vi "RUSHTarget.vi"(8 "Turret Case":i32, 9 "Joystick Value":dbl, 10 "Aspect Ratio":dbl[](array[numeric]), 11 "Target Info":T1(array[cluster])) -> (0 "Target Distance":dbl, 1 "Lock On Lights":i32, 3 "Raw Turret":dbl)   [LabVIEW 2011]
uses:
  GLOBALShooter.vi
panel:
  in  "Dead Band":dbl=0.09
  out "Offset":dbl
  in  "Minimum Power":dbl=0.22
  in  "Scale":dbl=0.85
  in  "AntiDrift":dbl
  out "Target X Coord":dbl
  out "Distance Array":dbl[](array[numeric])
  in  "Y AbsolVal Difference":dbl=0.25
  out "Number of Rectangles Visible":dbl
  out "Y Position Array":dbl[](array[numeric])
  out "X Position Array":dbl[](array[numeric])
  # "Settings"
  # "Inputs"
  # "Vision Info"
  # "Outputs"
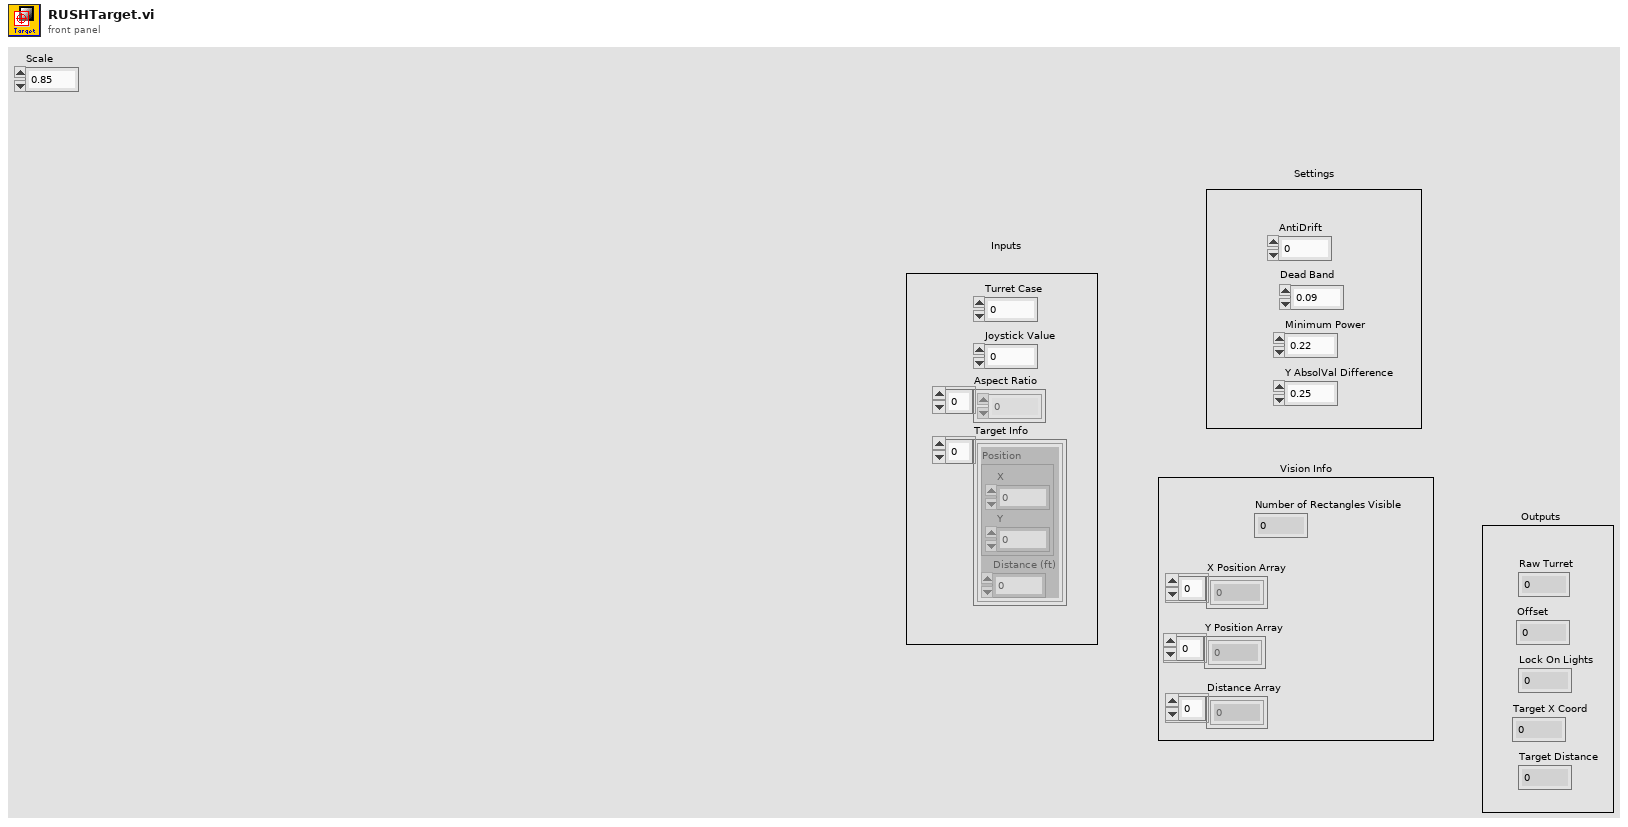
[diagram p1: front panel]
types:
  T1 = cluster{"Position":cluster{"X":dbl, "Y":dbl}, "Distance (ft)":dbl}[]
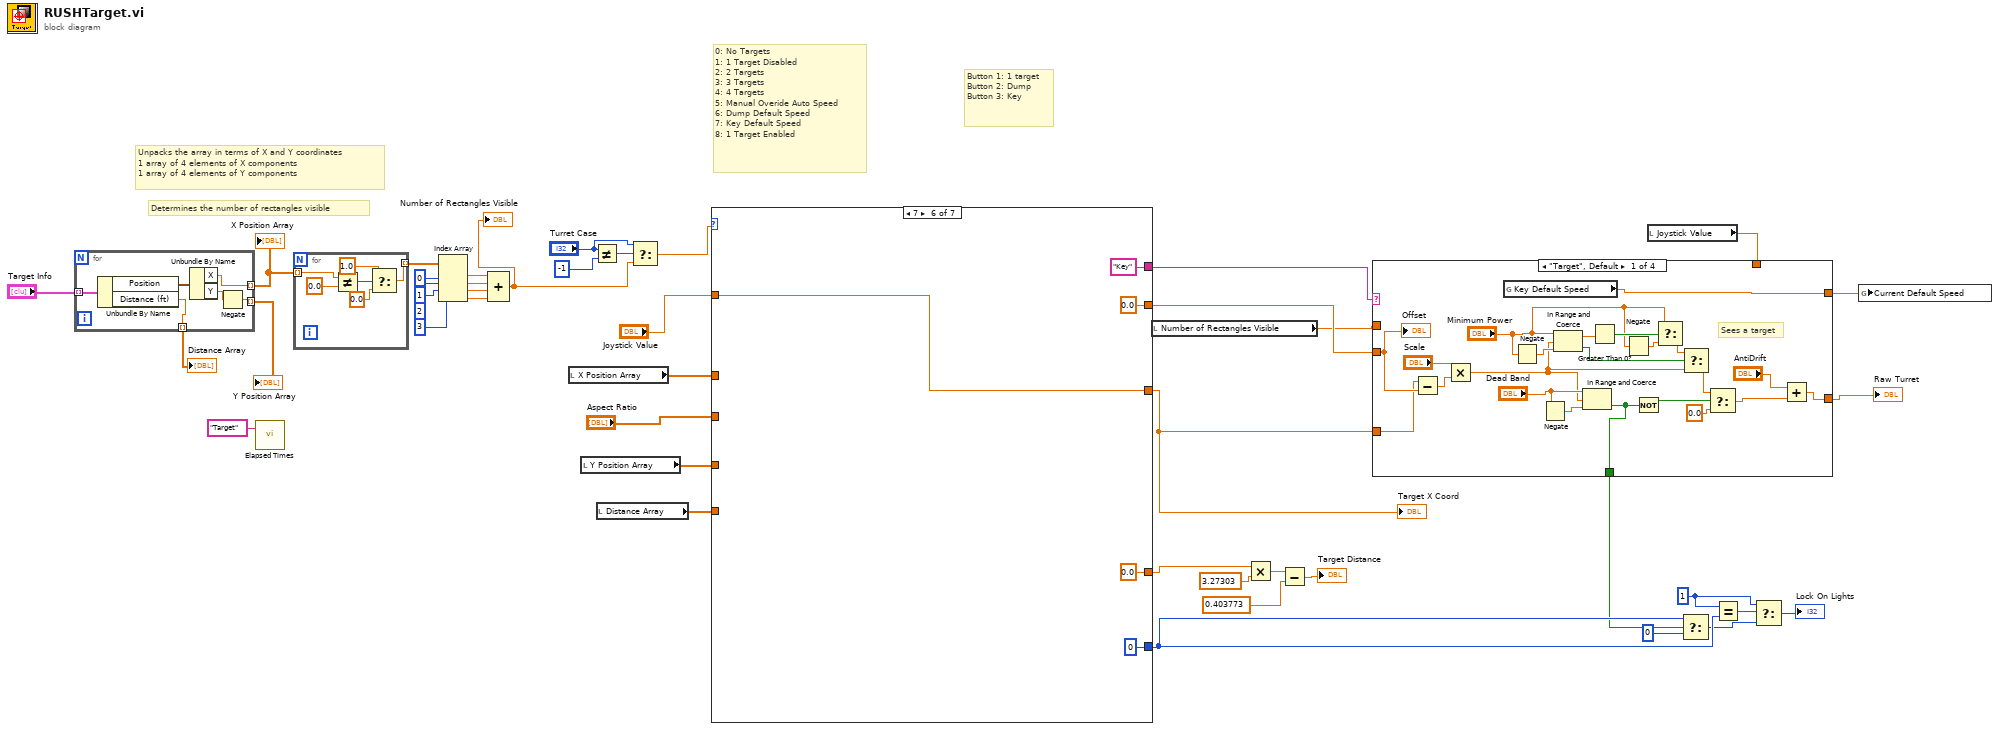
[diagram p0: block diagram]
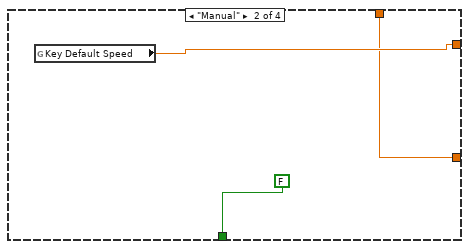
[diagram p2: hidden frame]
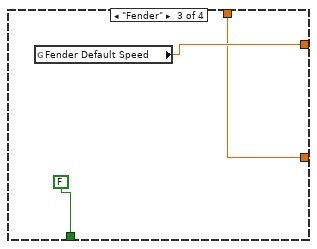
[diagram p3: hidden frame]
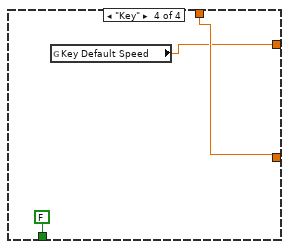
[diagram p4: hidden frame]
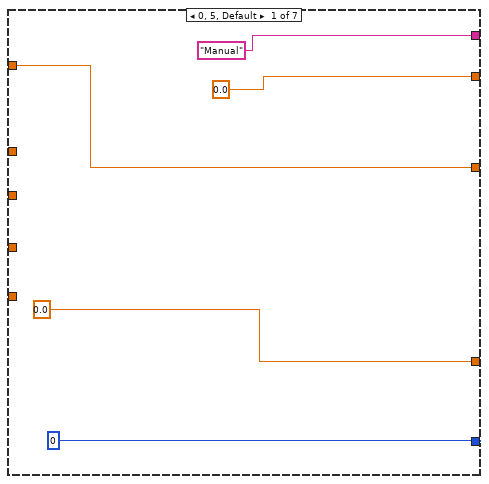
[diagram p5: hidden frame]
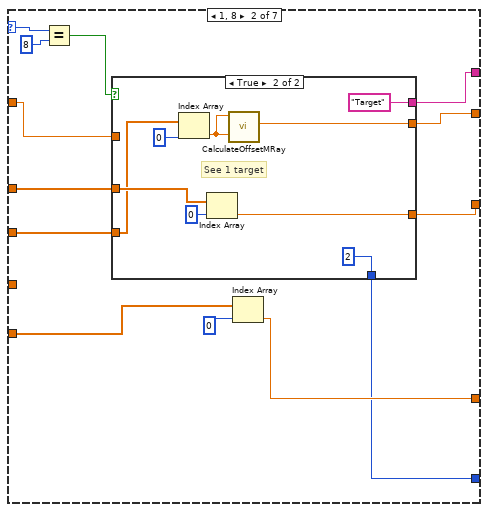
[diagram p6: hidden frame]
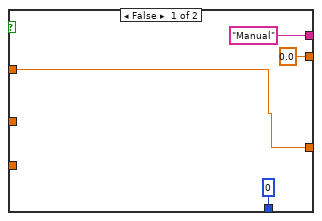
[diagram p7: hidden frame]
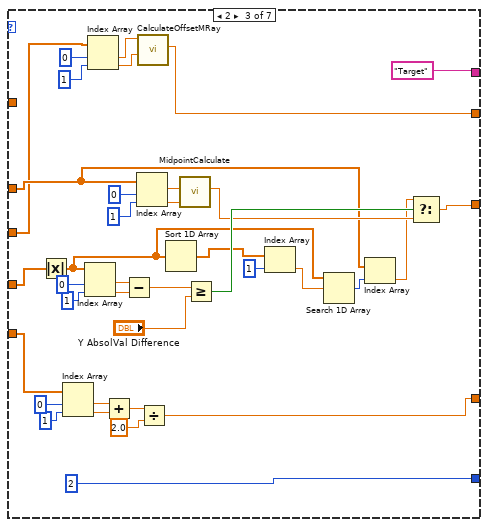
[diagram p8: hidden frame]
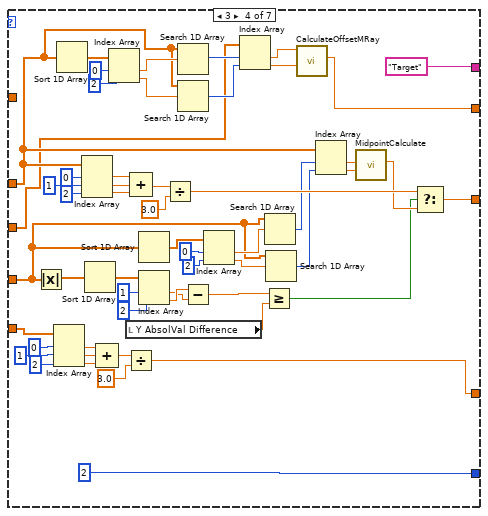
[diagram p9: hidden frame]
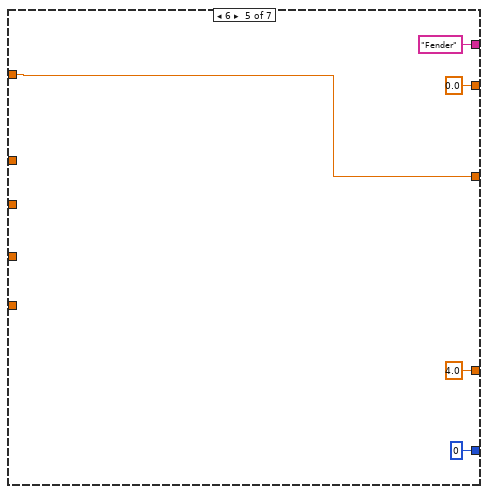
[diagram p10: hidden frame]
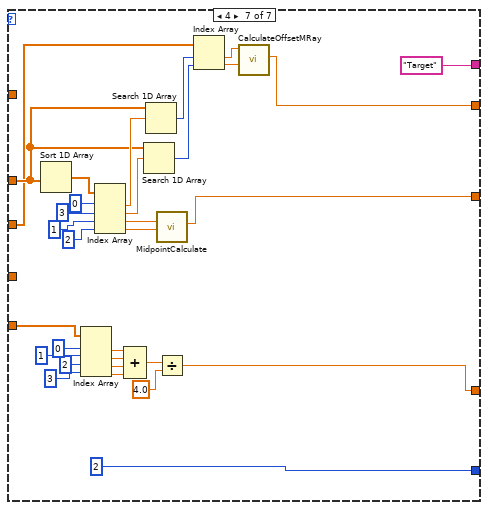
[diagram p11: hidden frame]
diagram:
  w26 = 1 ("y")
  # "Button 1: 1 target\nButton 2: Dump\nButton 3: Key"
  # "0: No Targets\n1: 1 Target Disabled\n2: 2 Targets\n3: 3 Targets\n4: 4 Targets\n5: Manual Overide Auto Speed\n6: Dump Default Speed\n7: Key Default Speed\n8: 1 Target Enabled"
  # "Determines the number of rectangles visible"
  # "Unpacks the array in terms of X and Y coordinates\n1 array of 4 elements of X components\n1 array of 4 elements of Y components"
  n1 = for {
    tunnel: [w47] -> w28 mode=indexing
    tunnel: [w48] -> w38 mode=indexing
    tunnel: "Target Info" -> [w45] mode=indexing
    tunnel: [w44] -> w40 mode=indexing
    n2 = Unbundle By Name(w45) -> ("Position"=w49:cluster{"X":dbl, "Y":dbl}, "Distance (ft)"=w44:dbl)
    n3 = Unbundle By Name(w49) -> ("X"=w48:dbl, "Y"=w46:dbl)
    n4 = Negate(x=w46) -> (-x=w47:dbl)
  }
  "X Position Array" <- w38
  "Y Position Array" <- w28
  "Distance Array" <- w40
  n5 = call "Elapsed Times.vi"("Call Name"="Target") -> ()  [unwired: 2 in, 1 out]
  n6 = for {
    tunnel: w38 -> [w54] mode=indexing
    tunnel: [w50] -> w37 mode=indexing
    n7 = Not Equal?(x=w54, y=0.0) -> (x != y?=w53:bool)
    n8 = Select(t=1.0, s=w53, f=0.0) -> (s? t:f=w50:dbl)
  }
  n9 = Index Array(array=w37, index #1=0 ("index"), index #2=1 ("index"), index #3=2 ("index"), index #4=3 ("index")) -> (element #1=w35:dbl, element #2=w36:dbl, element #3=w34:dbl, element #4=w33:dbl)
  n10 = Compound Arithmetic op=ADD(w35, w36, w34, w33) -> (w4:dbl)
  "Number of Rectangles Visible" <- w4
  n11 = local read "X Position Array"() -> (w39:dbl[])
  n12 = local read "Y Position Array"() -> (w41:dbl[])
  n13 = Not Equal?(x="Turret Case", y=-1) -> (x != y?=w6:bool)
  n14 = local read "Distance Array"() -> (w42:dbl[])
  n15 = Select(t="Turret Case", s=w6, f=w4) -> (s? t:f=w3:dbl)
  n16 = case shown="7" w3 {
    selector: w3 -> [_ w65 _ _ _ _ _]
    tunnel: w39 -> [_ w71 w92 w132 _ _ w194]
    tunnel: [w57 w70 w116 w166 w181 w185 w217] -> w21
    tunnel: w41 -> [_ _ w115 w144 _ _ _]
    tunnel: w42 -> [_ w68 w104 w175 _ _ w214]
    tunnel: [0 w66 2 2 0 0 2] -> w25
    tunnel: [0.0 ("Offset") w72 w121 w128 0.0 ("Offset") 0.0 ("Offset") w203] -> w22
    tunnel: "Aspect Ratio" -> [_ w73 w90 w127 _ _ w191]
    tunnel: [0.0 w67 w99 w168 4.0 ("X") 0.0 ("X") w204] -> w16
    tunnel: "Joystick Value" -> [w57 w62 _ _ w181 w185 _]
    tunnel: ["Manual" w61 "Target" "Target" "Fender" "Key" "Target"] -> w8
    frame 0, 5, Default {
    }
    frame 1, 8 {
      n17 = Equal?(x=w65, y=8) -> (x = y?=w63:bool)
      n18 = case shown="True" w63 {
        tunnel: w73 -> [_ w80]
        tunnel: [0.0 ("Offset") w85] -> w72
        tunnel: w71 -> [_ w83]
        tunnel: [w75 w82] -> w70
        tunnel: [0 2] -> w66
        tunnel: w62 -> [w75 _]
        tunnel: ["Manual" "Target"] -> w61
        frame False {
        }
        frame True {
          # "See 1 target"
          n19 = Index Array(array=w80, index=0) -> (element=w79:dbl)
          n20 = Index Array(array=w83, index=0) -> (element=w82:dbl)
          n21 = call "CalculateOffsetMRay.vi"("AR2"=w79, "AR1"=w79) -> ("Offset"=w85:dbl)  [unwired: 9 in]
        }
      }
      n22 = Index Array(array=w68, index=0) -> (element=w67:dbl)
    }
    frame 2 {
      n23 = Absolute Value(x=w115) -> (abs(x)=w95:dbl[])
      n24 = Index Array(array=w104, index #1=0 ("index"), index #2=1 ("index")) -> (element #1=w102:dbl, element #2=w103:dbl)
      n25 = Index Array(array=w95, index #1=0 ("index"), index #2=1 ("index")) -> (element #1=w111:dbl, element #2=w112:dbl)
      n26 = Index Array(array=w90, index #1=0 ("index"), index #2=1 ("index")) -> (element #1=w89:dbl, element #2=w88:dbl)
      n27 = Add(x=w102, y=w103) -> (x+y=w101:dbl)
      n28 = Subtract(x=w111, y=w112) -> (x-y=w110:dbl)
      n29 = Index Array(array=w92, index #1=0 ("index"), index #2=1 ("index")) -> (element #1=w117:dbl, element #2=w118:dbl)
      n30 = call "CalculateOffsetMRay.vi"("AR2"=w88, "AR1"=w89) -> ("Offset"=w121:dbl)  [unwired: 9 in]
      n31 = Divide(x=w101, y=2.0) -> (x/y=w99:dbl)
      n32 = Sort 1D Array(array=w95) -> (sorted array=w97:dbl[])
      n33 = call "MidpointCalculate.vi"("X2"=w118, "X1"=w117) -> ("Midpoint"=w107:dbl)  [unwired: 9 in]
      n34 = Greater Or Equal?(x=w110, y="Y AbsolVal Difference") -> (x >= y?=w108:bool)
      n35 = Index Array(array=w97, index=1) -> (element=w94:dbl)
      n36 = Search 1D Array(1D array=w95, element=w94) -> (index of element=w93:i32)  [unwired: 1 in]
      n37 = Index Array(array=w92, index=w93) -> (element=w91:dbl)
      n38 = Select(t=w91, s=w108, f=w107) -> (s? t:f=w116:dbl)
    }
    frame 3 {
      n39 = Absolute Value(x=w144) -> (abs(x)=w165:dbl[])
      n40 = Index Array(array=w175, index #1=0 ("index"), index #2=1 ("index"), index #3=2 ("index")) -> (element #1=w171:dbl, element #2=w172:dbl, element #3=w173:dbl)
      n41 = Sort 1D Array(array=w132) -> (sorted array=w136:dbl[])
      n42 = Index Array(array=w132, index #1=0 ("index"), index #2=1 ("index"), index #3=2 ("index")) -> (element #1=w153:dbl, element #2=w155:dbl, element #3=w154:dbl)
      n43 = Sort 1D Array(array=w165) -> (sorted array=w149:dbl[])
      n44 = Compound Arithmetic op=ADD(w171, w172, w173) -> (w170:dbl)
      n45 = Index Array(array=w136, index #1=0 ("index"), index #2=2 ("index")) -> (element #1=w133:dbl, element #2=w131:dbl)
      n46 = local read "Y AbsolVal Difference"() -> (w159:dbl)
      n47 = Divide(x=w170, y=3.0) -> (x/y=w168:dbl)
      n48 = Compound Arithmetic op=ADD(w153, w155, w154) -> (w152:dbl)
      n49 = Sort 1D Array(array=w144) -> (sorted array=w148:dbl[])
      n50 = Index Array(array=w149, index #1=1 ("index"), index #2=2 ("index")) -> (element #1=w161:dbl, element #2=w162:dbl)
      n51 = Divide(x=w152, y=3.0) -> (x/y=w150:dbl)
      n52 = Search 1D Array(1D array=w132, element=w133) -> (index of element=w130:i32)  [unwired: 1 in]
      n53 = Search 1D Array(1D array=w132, element=w131) -> (index of element=w129:i32)  [unwired: 1 in]
      n54 = Subtract(x=w162, y=w161) -> (x-y=w160:dbl)
      n55 = Index Array(array=w148, index #1=0 ("index"), index #2=2 ("index")) -> (element #1=w145:dbl, element #2=w143:dbl)
      n56 = Index Array(array=w127, index #1=w130, index #2=w129) -> (element #1=w126:dbl, element #2=w125:dbl)
      n57 = Greater Or Equal?(x=w160, y=w159) -> (x >= y?=w137:bool)
      n58 = Search 1D Array(1D array=w144, element=w145) -> (index of element=w142:i32)  [unwired: 1 in]
      n59 = Search 1D Array(1D array=w144, element=w143) -> (index of element=w141:i32)  [unwired: 1 in]
      n60 = call "CalculateOffsetMRay.vi"("AR2"=w125, "AR1"=w126) -> ("Offset"=w128:dbl)  [unwired: 9 in]
      n61 = Index Array(array=w132, index #1=w142, index #2=w141) -> (element #1=w139:dbl, element #2=w140:dbl)
      n62 = call "MidpointCalculate.vi"("X2"=w140, "X1"=w139) -> ("Midpoint"=w138:dbl)  [unwired: 9 in]
      n63 = Select(t=w150, s=w137, f=w138) -> (s? t:f=w166:dbl)
    }
    frame 6 {
    }
    frame 7 {
    }
    frame 4 {
      n64 = Sort 1D Array(array=w194) -> (sorted array=w218:dbl[])
      n65 = Index Array(array=w214, index #1=0 ("index"), index #2=1 ("index"), index #3=2 ("index"), index #4=3 ("index")) -> (element #1=w211:dbl, element #2=w210:dbl, element #3=w209:dbl, element #4=w208:dbl)
      n66 = Index Array(array=w218, index #1=0 ("index"), index #2=3 ("index"), index #3=1 ("index"), index #4=2 ("index")) -> (element #1=w195:dbl, element #2=w196:dbl, element #3=w202:dbl, element #4=w201:dbl)
      n67 = Compound Arithmetic op=ADD(w211, w210, w209, w208) -> (w207:dbl)
      n68 = Search 1D Array(1D array=w194, element=w196) -> (index of element=w193:i32)  [unwired: 1 in]
      n69 = Search 1D Array(1D array=w194, element=w195) -> (index of element=w192:i32)  [unwired: 1 in]
      n70 = call "MidpointCalculate.vi"("X2"=w201, "X1"=w202) -> ("Midpoint"=w217:dbl)  [unwired: 9 in]
      n71 = Divide(x=w207, y=4.0) -> (x/y=w204:dbl)
      n72 = Index Array(array=w191, index #1=w192, index #2=w193) -> (element #1=w190:dbl, element #2=w189:dbl)
      n73 = call "CalculateOffsetMRay.vi"("AR2"=w189, "AR1"=w190) -> ("Offset"=w203:dbl)  [unwired: 9 in]
    }
  }
  "Target X Coord" <- w21
  n74 = local read "Number of Rectangles Visible"() -> (w9:dbl)
  n75 = Multiply(x=w16, y=3.27303) -> (x*y=w19:dbl)
  n76 = Subtract(x=w19, y=0.403773) -> (x-y=→"Target Distance":dbl)
  n77 = local read "Joystick Value"() -> (w10:dbl)
  n78 = case shown="\"Target\", Default" w8 {
    tunnel: w22 -> [w239 _ _ _]
    tunnel: w21 -> [w238 _ _ _]
    tunnel: [w221 w241 w244 w249] -> w1
    tunnel: [w224 FALSE FALSE FALSE] -> w20
    tunnel: w9 -> [_ _ _ _]
    tunnel: w10 -> [_ w241 w244 w249]
    tunnel: [w219 w242 w245 w247] -> w2
    frame "Target", Default {
      # "Sees a target"
      n79 = Subtract(x=w238, y=w239) -> (x-y=w236:dbl)
      n80 = Multiply(x="Scale", y=w236) -> (x*y=w227:dbl)
      n81 = global read "GLOBALShooter.vi" "Key Default Speed"() -> (w219:dbl)
      n82 = Negate(x="Minimum Power") -> (-x=w234:dbl)
      n83 = Negate(x="Dead Band") -> (-x=w240:dbl)
      n84 = In Range and Coerce(upper limit="Minimum Power", x=w227, lower limit=w234) -> (coerced(x)=w230:dbl, In Range?=w231:bool)
      n85 = In Range and Coerce(upper limit="Dead Band", x=w227, lower limit=w240) -> (In Range?=w224:bool)  [unwired: 1 out]
      n86 = Greater Than 0?(x=w230) -> (x > 0?=w229:bool)
      n87 = Negate(x="Minimum Power") -> (-x=w226:dbl)
      n88 = Not(x=w224) -> (.not. x?=w225:bool)
      n89 = Select(t="Minimum Power", s=w229, f=w226) -> (s? t:f=w228:dbl)
      n90 = Select(t=w228, s=w231, f=w227) -> (s? t:f=w232:dbl)
      n91 = Select(t=w232, s=w225, f=0.0) -> (s? t:f=w222:dbl)
      n92 = Add(x="AntiDrift", y=w222) -> (x+y=w221:dbl)
      "Offset" <- w239
    }
    frame "Manual" {
      n93 = global read "GLOBALShooter.vi" "Key Default Speed"() -> (w242:dbl)
    }
    frame "Fender" {
      n94 = global read "GLOBALShooter.vi" "Fender Default Speed"() -> (w245:dbl)
    }
    frame "Key" {
      n95 = global read "GLOBALShooter.vi" "Key Default Speed"() -> (w247:dbl)
    }
  }
  "Raw Turret" <- w1
  n96 = Select(t=w25, s=w20, f=0) -> (s? t:f=w23:i32)
  n97 = Equal?(x=w26, y=w25) -> (x = y?=w27:bool)
  n98 = Select(t=w26, s=w27, f=w23) -> (s? t:f=→"Lock On Lights":i32)
  n99 = global write "GLOBALShooter.vi" "Current Default Speed"(w2) -> ()
